vi "SL2_AD_DLL_Phoibos_Terminate.vi"(4 "error in":errorcluster, 7 "dll path in":path) -> (0 "error out":errorcluster, 3 "dll path out":path)   [LabVIEW 2020]
panel:
  out "error out 2":errorcluster
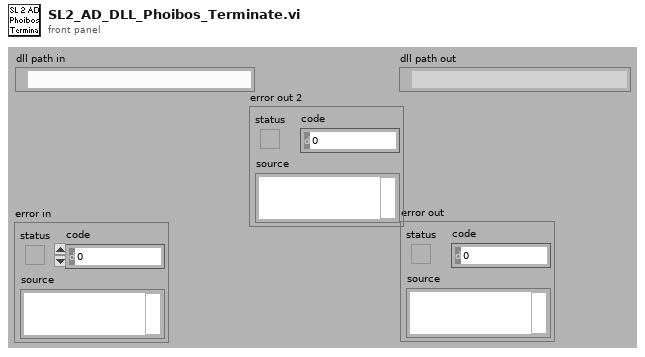
[diagram p1: front panel]
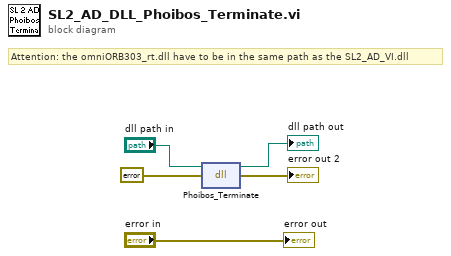
[diagram p0: block diagram]
diagram:
  # "Attention: the omniORB303_rt.dll have to be in the same path as the SL2_AD_VI.dll"
  n1 = dll-call lib="C:/Programme/SPECS/SpecsLab2/programming/LabView7.1/SL2_AD_VI.dll" fn="Phoibos_Terminate"(path in="dll path in", error in=errorcluster {"status"=FALSE, "code"=0, "source"=""} ("error out")) -> (path out=→"dll path out":path, error out=→"error out 2":errorcluster)  [unwired: 2 in]
  "error out" <- "error in"
